vi "Crack.vi"() -> ()   [LabVIEW 2011]
uses:
  C:/Program Files (x86)/National Instruments/LabVIEW 2011/resource/objmgr/daqmx.rc
panel:
  in  "Crack":bool
  in  "注册文件路径":path=path "D:/开关测试/Config/Reg.dat"
  in  "R/W":enum16{"R", "W"}(ring)=enum."W"
  # "注册系统"
  # "用于电器开关通用测试台系统注册。\nEnjoy it!"
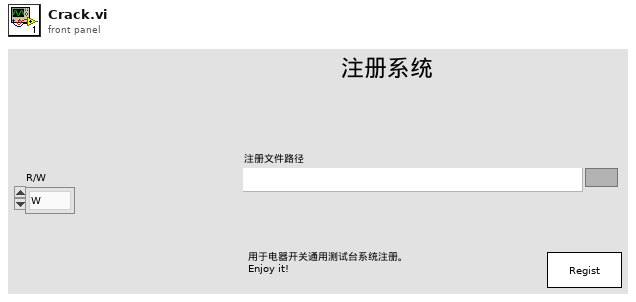
[diagram p1: front panel]
types:
  T1 = enum16{"open", "replace", "create", "open or create", "replace or create", "replace or create with confirmation"}
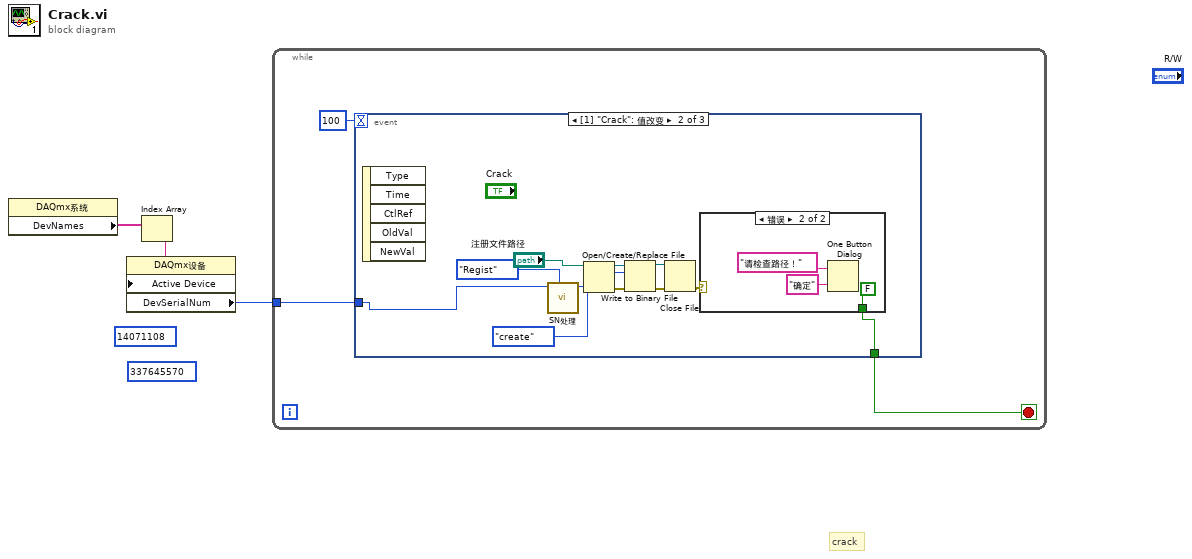
[diagram p0: block diagram]
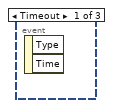
[diagram p2: hidden frame]
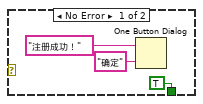
[diagram p3: hidden frame]
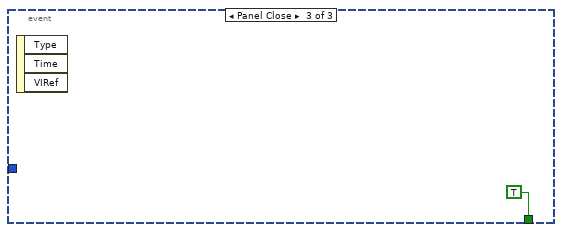
[diagram p4: hidden frame]
diagram:
  (unwired) 14071108 ("SN号")
  (unwired) 337645570 ("SN号")
  # "crack"
  n1 = property class="DAQmx系统"() -> ("DevNames"=w2:tag[])  [unwired: 2 in, 2 out]
  n2 = Index Array(array=w2) -> (element=w1:tag)  [unwired: 1 in]
  n3 = property class="DAQmx设备"("Active Device"=w1) -> ("DevSerialNum"=w3:u32)  [unwired: 2 in, 2 out]
  n4 = while {
    tunnel: w3 -> [w4]
    stop <- w5 stop-if-true
    n5 = event shown="[1] \"Crack\": 值改变" {
      selector: _ -> [_ _ _]
      dyn-events: _ -> [_ _ _]
      timeout: 100 -> [_ _ _]
      tunnel: [_ w12 TRUE] -> w5
      tunnel: w4 -> [_ w7 _]
      event Timeout {
        n6 = event-data() -> ()  [unwired: 1 in, 2 out]
      }
      event "Crack": Value Change {
        n7 = event-data() -> ()  [unwired: 1 in, 5 out]
        n8 = call "SN处理.vi"("动作"=enum16{"Check", "Regist"}."Regist", "SN号"=w7) -> ("SN"=w17:u32)  [unwired: 9 in]
        n9 = Open/Create/Replace File(file path (use dialog)="注册文件路径", operation (0:open)=T1."create" ("操作(0:open)")) -> (refnum out=w11:refnum<file>, error out=w10:errorcluster)  [unwired: 4 in, 1 out]
        n10 = Write to Binary File(file (use dialog)=w11, data=w17, error in=w10) -> (refnum out=w16:refnum<file>, error out=w15:errorcluster)  [unwired: 3 in, 1 out]
        n11 = Close File(refnum=w16, error in=w15) -> (error out=w13:errorcluster)  [unwired: 1 out]
        n12 = case shown="错误" w13 {
          tunnel: [TRUE FALSE] -> w12
          frame No Error {
            n13 = One Button Dialog(message="注册成功！" ("消息"), button name ("OK")="确定" ("按钮名称（“确定”）")) -> ()  [unwired: 1 out]
          }
          frame Error {
            n14 = One Button Dialog(message="请检查路径！" ("消息"), button name ("OK")="确定" ("按钮名称（“确定”）")) -> ()  [unwired: 1 out]
          }
        }
      }
      event Panel Close {
        n15 = event-data() -> ()  [unwired: 1 in, 3 out]
      }
    }
  }
